vi "Configure Trigger.vi"(4 "Pacing Time (0.02)":dbl=0.02 min=2e-06 max=500.0, 6 "Pacing State (F: Off)":bool, 7 "Hold Off State (T: On)":bool=TRUE, 8 "error in (no error)":errorcluster, 9 "Hold Off Time (0.0002)":dbl=0.0002, 10 "Trigger Count (1)":i32=1, 11 "VISA resource name":refnum<visa-resource-name>) -> (0 "error out":errorcluster, 3 "VISA resource name out":refnum<visa-resource-name>)   [LabVIEW 2019, in "Pendulum CNT90.lvlib"]
doc: "Configures edge trigger settings. Sets how many measurements the instrument should make for each arming start. Switches the Hold Off function On/Off and sets the Hold Off time value."
uses:
  Pendulum CNT90.lvlib
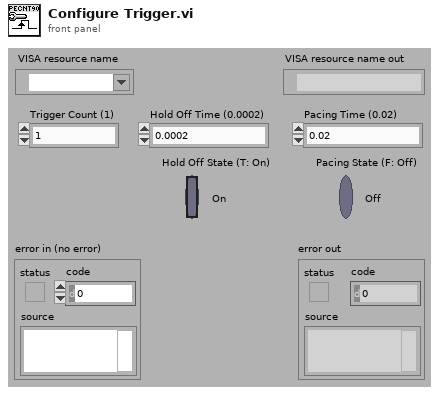
[diagram p1: front panel]
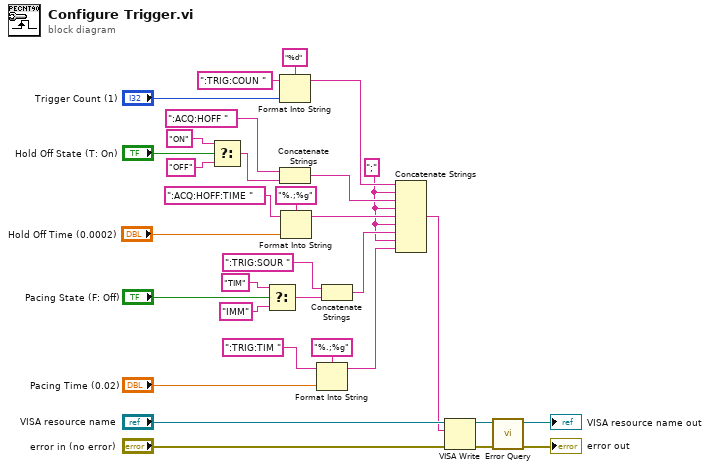
[diagram p0: block diagram]
diagram:
  w2 = ";"
  n1 = Select(t="ON", s="Hold Off State (T: On)", f="OFF") -> (s? t:f=w20:string)
  n2 = Select(t="TIM", s="Pacing State (F: Off)", f="IMM") -> (s? t:f=w9:string)
  n3 = Format Into String(format string="%d", initial string=":TRIG:COUN " ("format string"), "Trigger Count (1)") -> (resulting string=w13:string)  [unwired: 1 in, 1 out]
  n4 = Concatenate Strings(":ACQ:HOFF ", w20) -> (w15:string)
  n5 = Format Into String(format string="%.;%g", initial string=":ACQ:HOFF:TIME ", "Hold Off Time (0.0002)") -> (resulting string=w14:string)  [unwired: 1 in, 1 out]
  n6 = Format Into String(format string="%.;%g", initial string=":TRIG:TIM ", "Pacing Time (0.02)") -> (resulting string=w1:string)  [unwired: 1 in, 1 out]
  n7 = Concatenate Strings(":TRIG:SOUR ", w9) -> (w3:string)
  n8 = Concatenate Strings(w13, w2, w15, w2, w14, w2, w3, w2, w1) -> (w12:string)
  n9 = VISA Write(VISA resource name="VISA resource name", write buffer=w12, error in (no error)="error in (no error)") -> (VISA resource name out=w28:refnum<visa-resource-name>, error out=w27:errorcluster)  [unwired: 1 out]
  n10 = call "Error Query.vi"("error in (no error)"=w27, "VISA resource name"=w28) -> ("error out"=→"error out":errorcluster, "VISA resource name out"=→"VISA resource name out":refnum<visa-resource-name>)  [unwired: 6 in, 2 out]
